vi "Initialize Topics.vi"(11 "Functions":T2=[0, 8, 12]) -> (0 "error out":errorcluster)   [LabVIEW 2013]
uses:
  Functions.ctl
  ROS/Code/SubVIs/BaxterSide.ctl
  ROS/Code/SubVIs/BaxterButtons.ctl
  ROS/Code/SubVIs/BaxterCamera.ctl
  BaxterVIs/Read_Joint_States_A.vi
panel:
  in  "Enable Only":bool
  in  "Run Segmenter 2":bool=TRUE
  out "Cameras List":T1
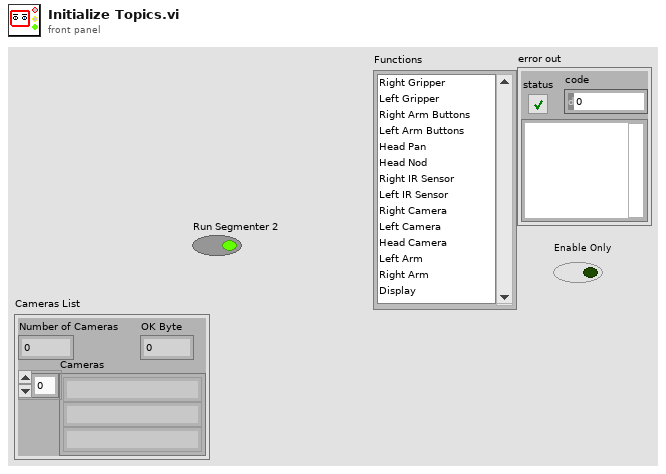
[diagram p1: front panel]
types:
  T1 = cluster{"Number of Cameras":i32, "Cameras":string[], "OK Byte":u8}
  T2 = typedef "Functions.ctl" = i32[]
  T3 = typedef "BaxterSide.ctl" = enum16{"left", "right"}
  T4 = typedef "BaxterCamera.ctl" = enum16{"left_hand_camera", "right_hand_camera", "head_camera"}
  T5 = cluster{"Camera":T4, "FPS":sgl, "Camera Controls":cluster{"id":i32, "value":i32}[], "Resolution":enum16{"(1280, 800)", "(960, 600)", "(640, 400)", "(480, 300)", "(384, 240)", "(320, 200)"}}
  T6 = cluster{"Label":string, "Arm Angles (degrees)":dbl[]}
  T7 = typedef "BaxterButtons.ctl" = u16
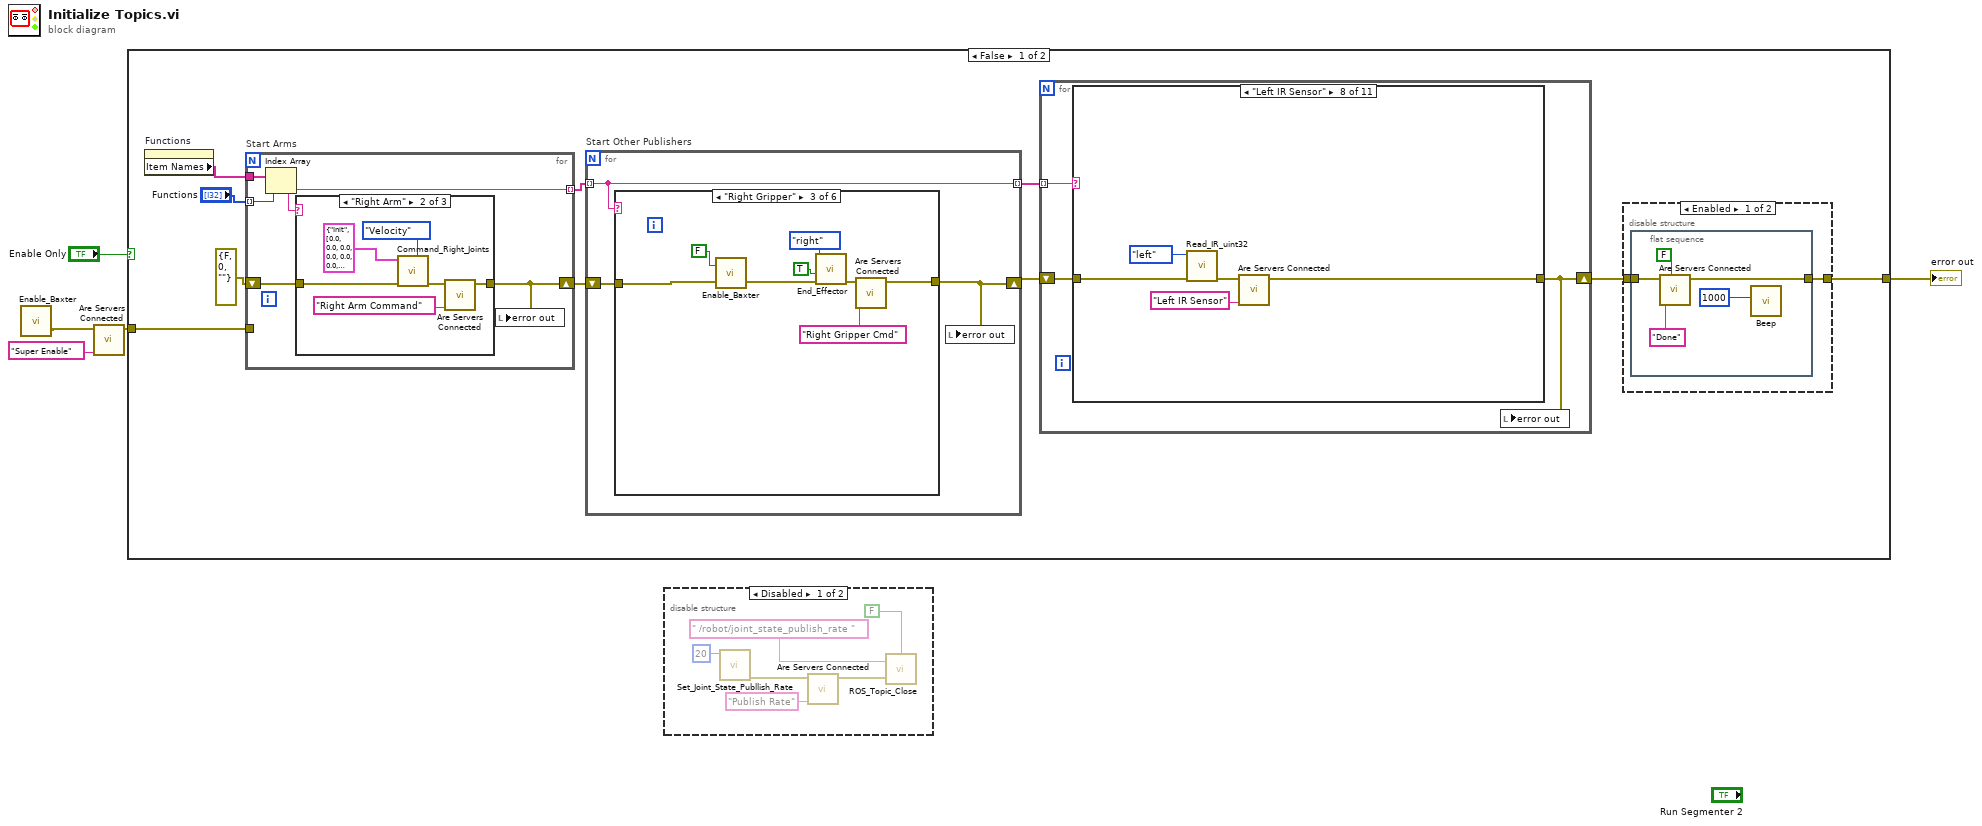
[diagram p0: block diagram]
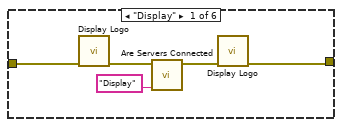
[diagram p2: hidden frame]
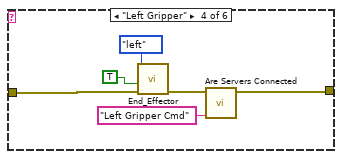
[diagram p4: hidden frame]
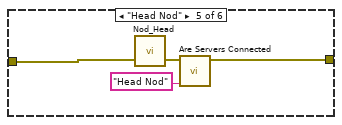
[diagram p5: hidden frame]
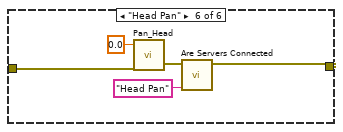
[diagram p6: hidden frame]
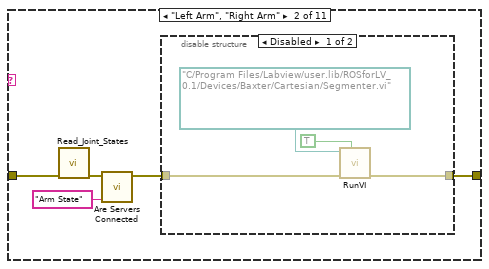
[diagram p9: hidden frame]
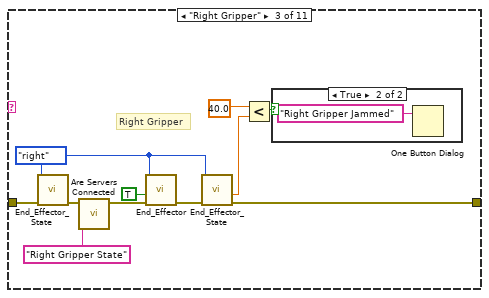
[diagram p11: hidden frame]
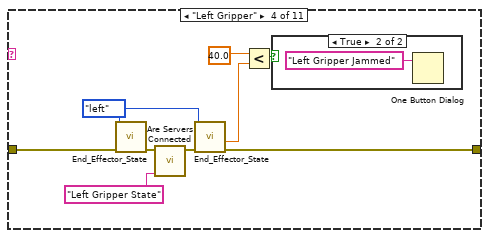
[diagram p13: hidden frame]
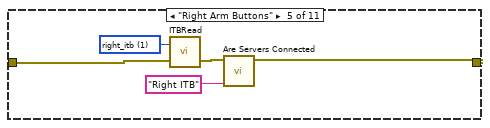
[diagram p15: hidden frame]
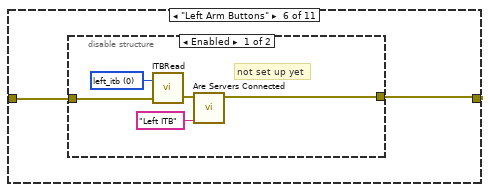
[diagram p16: hidden frame]
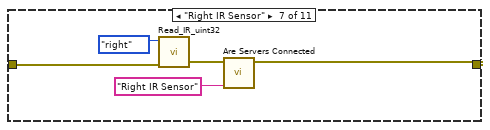
[diagram p18: hidden frame]
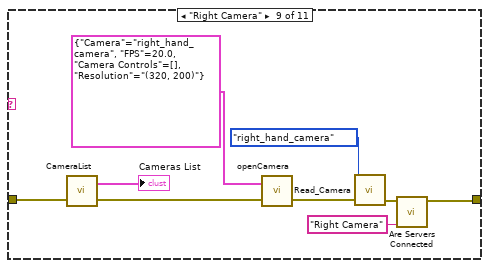
[diagram p19: hidden frame]
diagram:
  n1 = call "Enable_Baxter.vi"() -> ("error out"=w4:errorcluster)  [unwired: 4 in]
  n2 = call "Are Servers Connected.vi"("Activity"="Super Enable", "error in"=w4) -> ("error out"=w2:errorcluster)  [unwired: 6 in, 1 out]
  n3 = case shown="False" "Enable Only" {
    tunnel: [w8 w145] -> w3
    tunnel: w2 -> [w6 w145]
    frame False {
      n4 = property on="Functions" class="LstBox (strict)"() -> ("Item Names"=w14:string[])  [unwired: 2 in, 2 out]
      n5 = for "Start Arms" {
        tunnel: "Functions" -> [w128] mode=indexing
        shift-right: [w126] -> w10
        shift-left: errorcluster {"status"=FALSE, "code"=0, "source"=""} ("error out") -> [w130]
        tunnel: w14 -> [w129]
        tunnel: [w127] -> w13 mode=indexing
        tunnel: w6 -> [_]
        n6 = Index Array(array=w129, index=w128) -> (element=w127:string)
        n7 = case shown="\"Right Arm\"" w127 {
          tunnel: w130 -> [w131 w133 w140]
          tunnel: [w131 w136 w142] -> w126
          frame Default {
          }
          frame "Right Arm" {
            n8 = call "Command_Right_Joints.vi"("Mode"=enum32{"Position", "Velocity", "Effort"}."Velocity", "error in"=w133, "Goal"=T6 {"Label"="Init", "Arm Angles (degrees)"=[0.0, 0.0, 0.0, 0.0, 0.0, 0.0, 0.0]}) -> ("error out"=w132:errorcluster)  [unwired: 5 in, 1 out]
            n9 = call "Are Servers Connected.vi"("Activity"="Right Arm Command", "error in"=w132) -> ("error out"=w136:errorcluster)  [unwired: 6 in, 1 out]
          }
          frame "Left Arm" {
            n10 = call "Command_Left_Joints.vi"("Mode"=enum32{"Position", "Velocity", "Effort"}."Velocity", "error in"=w140, "Goal"=T6 {"Label"="Init", "Arm Angles (degrees)"=[0.0, 0.0, 0.0, 0.0, 0.0, 0.0, 0.0]}) -> ("error out"=w139:errorcluster)  [unwired: 5 in, 1 out]
            n11 = call "Are Servers Connected.vi"("Activity"="Left Arm Command", "error in"=w139) -> ("error out"=w142:errorcluster)  [unwired: 6 in, 1 out]
          }
        }
        n12 = local write "error out"(w126) -> ()
      }
      n13 = for "Start Other Publishers" {
        shift-right: [w16] -> w11
        shift-left: w10 -> [w18]
        tunnel: [w17] -> w12 mode=indexing
        tunnel: w13 -> [w17] mode=indexing
        n14 = case shown="\"Right Gripper\"" w17 {
          tunnel: w18 -> [w22 w24 w27 w33 w40 w44]
          tunnel: [w19 w24 w28 w38 w39 w43] -> w16
          frame "Display" {
            n15 = call "Display Logo.vi"("error in"=w22) -> ("error out"=w21:errorcluster)  [unwired: 10 in]
            n16 = call "Are Servers Connected.vi"("Activity"="Display", "error in"=w21) -> ("error out"=w20:errorcluster)  [unwired: 6 in, 1 out]
            n17 = call "Display Logo.vi"("error in"=w20) -> ("error out"=w19:errorcluster)  [unwired: 10 in]
          }
          frame Default {
          }
          frame "Right Gripper" {
            n18 = call "Enable_Baxter.vi"("error in"=w27, "Enable?"=FALSE) -> ("error out"=w26:errorcluster)  [unwired: 2 in]
            n19 = call "End_Effector.vi"("error in"=w26, "Calibrate"=TRUE, "Side"=BaxterSide."right") -> ("error out"=w29:errorcluster)  [unwired: 5 in]
            n20 = call "Are Servers Connected.vi"("Activity"="Right Gripper Cmd", "error in"=w29) -> ("error out"=w28:errorcluster)  [unwired: 6 in, 1 out]
          }
          frame "Left Gripper" {
            n21 = call "End_Effector.vi"("error in"=w33, "Calibrate"=TRUE, "Side"=BaxterSide."left") -> ("error out"=w35:errorcluster)  [unwired: 5 in]
            n22 = call "Are Servers Connected.vi"("Activity"="Left Gripper Cmd", "error in"=w35) -> ("error out"=w38:errorcluster)  [unwired: 6 in, 1 out]
          }
          frame "Head Nod" {
            n23 = call "Nod_Head.vi"("error in"=w40) -> ("error out"=w41:errorcluster)  [unwired: 3 in]
            n24 = call "Are Servers Connected.vi"("Activity"="Head Nod", "error in"=w41) -> ("error out"=w39:errorcluster)  [unwired: 6 in, 1 out]
          }
          frame "Head Pan" {
            n25 = call "Pan_Head.vi"("error in"=w44, "target"=sgl 0.0) -> ("error out"=w46:errorcluster)  [unwired: 3 in]
            n26 = call "Are Servers Connected.vi"("Activity"="Head Pan", "error in"=w46) -> ("error out"=w43:errorcluster)  [unwired: 6 in, 1 out]
          }
        }
        n27 = local write "error out"(w16) -> ()
      }
      n28 = for {
        shift-right: [w56] -> w9
        shift-left: w11 -> [w58]
        tunnel: w12 -> [w57] mode=indexing
        n29 = case shown="\"Left IR Sensor\"" w57 {
          tunnel: w58 -> [w59 w62 w78 w88 w93 w98 w106 w111 w123 w124 w125]
          tunnel: [w59 w60 w76 w84 w92 w97 w105 w110 w121 w124 w125] -> w56
          frame Default {
          }
          frame "Left Arm", "Right Arm" {
            n30 = call-poly "Read_Joint_States.vi"("error in"=w62) -> ("error out"=w63:errorcluster)  [unwired: 4 in, 3 out]
            n31 = call "Are Servers Connected.vi"("Activity"="Arm State", "error in"=w63) -> ("error out"=w61:errorcluster)  [unwired: 6 in, 1 out]
            n32 = disable-structure shown="Disabled" {
              disable-tunnel: w61 -> [w66 w69]
              disable-tunnel: [w65 w69] -> w60
              frame Disabled {
                n33 = call "RunVI.vi"("Visible?"=TRUE, "error in"=w66, "vi path"=path "C:/Program Files/Labview/user.lib/ROSforLV_0.1/Devices/Baxter/Cartesian/Segmenter.vi") -> ("error out"=w65:errorcluster)  [unwired: 6 in]
              }
              frame Enabled {
              }
            }
          }
          frame "Right Gripper" {
            w71 = BaxterSide."right" ("Side")
            # "Right Gripper"
            n34 = call "End_Effector_State.vi"("error in"=w78, "Side"=w71) -> ("error out"=w79:errorcluster)  [unwired: 3 in, 3 out]
            n35 = call "Are Servers Connected.vi"("Activity"="Right Gripper State", "error in"=w79) -> ("error out"=w73:errorcluster)  [unwired: 6 in, 1 out]
            n36 = call "End_Effector.vi"("error in"=w73, "Calibrate"=TRUE, "Side"=w71) -> ("error out"=w72:errorcluster)  [unwired: 5 in]
            n37 = call "End_Effector_State.vi"("error in"=w72, "Side"=w71) -> ("error out"=w76:errorcluster, "force"=w74:sgl)  [unwired: 3 in, 2 out]
            n38 = Less?(x=sgl 40.0 ("y"), y=w74) -> (x < y?=w77:bool)
            n39 = case shown="True" w77 {
              frame False {
              }
              frame True {
                n40 = One Button Dialog(message="Right Gripper Jammed") -> ()  [unwired: 1 in, 1 out]
              }
            }
          }
          frame "Left Gripper" {
            w86 = BaxterSide."left" ("Side")
            n41 = call "End_Effector_State.vi"("error in"=w88, "Side"=w86) -> ("error out"=w89:errorcluster)  [unwired: 3 in, 3 out]
            n42 = call "Are Servers Connected.vi"("Activity"="Left Gripper State", "error in"=w89) -> ("error out"=w87:errorcluster)  [unwired: 6 in, 1 out]
            n43 = call "End_Effector_State.vi"("error in"=w87, "Side"=w86) -> ("error out"=w84:errorcluster, "force"=w82:sgl)  [unwired: 3 in, 2 out]
            n44 = Less?(x=sgl 40.0 ("y"), y=w82) -> (x < y?=w85:bool)
            n45 = case shown="True" w85 {
              frame False {
              }
              frame True {
                n46 = One Button Dialog(message="Left Gripper Jammed") -> ()  [unwired: 1 in, 1 out]
              }
            }
          }
          frame "Right Arm Buttons" {
            w96 = T7 1 items=["left_itb", "right_itb", "torso_left_itb", "torso_right_itb"] ("Component")
            n47 = call "ITBRead.vi"("error in"=w93, "Component"=w96) -> ("error out"=w94:errorcluster)  [unwired: 1 in, 1 out]
            n48 = call "Are Servers Connected.vi"("Activity"="Right ITB", "error in"=w94) -> ("error out"=w92:errorcluster)  [unwired: 6 in, 1 out]
          }
          frame "Left Arm Buttons" {
            n49 = disable-structure shown="Enabled" {
              disable-tunnel: w98 -> [w100 w104]
              disable-tunnel: [w99 w104] -> w97
              frame Enabled {
                w103 = T7 0 items=["left_itb", "right_itb", "torso_left_itb", "torso_right_itb"] ("Component")
                # "not set up yet"
                n50 = call "ITBRead.vi"("error in"=w100, "Component"=w103) -> ("error out"=w101:errorcluster)  [unwired: 1 in, 1 out]
                n51 = call "Are Servers Connected.vi"("Activity"="Left ITB", "error in"=w101) -> ("error out"=w99:errorcluster)  [unwired: 6 in, 1 out]
              }
              frame Disabled {
              }
            }
          }
          frame "Right IR Sensor" {
            n52 = call "Read_IR_uint32.vi"("error in"=w106, "Side"=BaxterSide."right") -> ("error out"=w107:errorcluster)  [unwired: 3 in, 3 out]
            n53 = call "Are Servers Connected.vi"("Activity"="Right IR Sensor", "error in"=w107) -> ("error out"=w105:errorcluster)  [unwired: 6 in, 1 out]
          }
          frame "Left IR Sensor" {
            n54 = call "Read_IR_uint32.vi"("error in"=w111, "Side"=BaxterSide."left") -> ("error out"=w112:errorcluster)  [unwired: 3 in, 3 out]
            n55 = call "Are Servers Connected.vi"("Activity"="Left IR Sensor", "error in"=w112) -> ("error out"=w110:errorcluster)  [unwired: 6 in, 1 out]
          }
          frame "Right Camera" {
            n56 = call "CameraList.vi"("error in"=w123) -> ("error out"=w122:errorcluster, "Cameras List"=→"Cameras List":T1)  [unwired: 1 in]
            n57 = call "openCamera.vi"("error in"=w122, "Camera Settings"=T5 {"Camera"=enum."right_hand_camera", "FPS"=20.0, "Camera Controls"=[], "Resolution"=enum."(320, 200)"}) -> ("error out"=w118:errorcluster)  [unwired: 1 in, 1 out]
            n58 = call "Read_Camera.vi"("Camera"=BaxterCamera."right_hand_camera", "error in"=w118) -> ("error out"=w117:errorcluster)  [unwired: 1 in, 4 out]
            n59 = call "Are Servers Connected.vi"("Activity"="Right Camera", "error in"=w117) -> ("error out"=w121:errorcluster)  [unwired: 6 in, 1 out]
          }
          frame "Left Camera" {
          }
          frame "Head Camera" {
          }
        }
        n60 = local write "error out"(w56) -> ()
      }
      n61 = disable-structure shown="Enabled" {
        disable-tunnel: w9 -> [w49 w55]
        disable-tunnel: [w48 w55] -> w8
        frame Enabled {
          n62 = flat-sequence {
            tunnel: w49 -> [w52]
            tunnel: [w51] -> w48
            frame #0 {
              n63 = call "Are Servers Connected.vi"("Wait"=FALSE, "Activity"="Done", "error in"=w52) -> ("error out"=w51:errorcluster)  [unwired: 5 in, 1 out]
              n64 = call <vilib>:"Beep.vi"("duration (msec)"=u32 1000) -> ()  [unwired: 11 in]
            }
          }
        }
        frame Disabled {
        }
      }
    }
    frame True {
      n65 = local write "Enable Only"(FALSE ("Enable Only")) -> ()
    }
  }
  "error out" <- w3
  n66 = disable-structure shown="Disabled" {
    frame Disabled {
      n67 = call "Set_Joint_State_Publlish_Rate.vi"("Publish Rate"=u32 20) -> ("error out"=w149:errorcluster)  [unwired: 8 in]
      n68 = call "Are Servers Connected.vi"("Activity"="Publish Rate", "error in"=w149) -> ("error out"=w148:errorcluster)  [unwired: 6 in, 1 out]
      n69 = call "ROS_Topic_Close.vi"("error in"=w148, "topic"=" /robot/joint_state_publish_rate ", "StopConsole"=FALSE) -> ()  [unwired: 1 in, 1 out]
    }
    frame Enabled {
    }
  }
